vi "Create Enum Type Specialization.vi"(7 "error in":errorcluster, 9 "parameter name":string, 10 "enum reference in":refnum<vi>) -> (0 "error out":errorcluster, 2 "parameter type specialization output":T1, 3 "control reference out":refnum<vi>)   [LabVIEW 2020, in "Measurement Plugin Measurement Server.lvlib"]
uses:
  Measurement Plugin Measurement Server.lvlib
  TypeDefs/Parameter Type Specialization.ctl
  TypeDefs/Type Specialization.ctl
  TypeDefs/Type Specialization Key.ctl
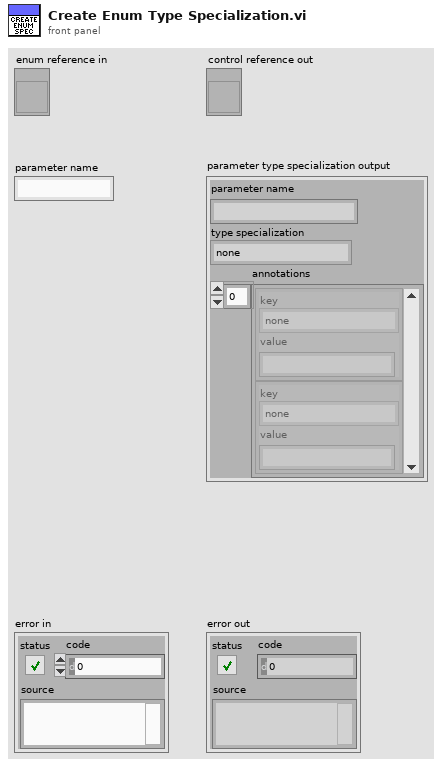
[diagram p1: front panel]
types:
  T1 = typedef "Measurement Plugin Measurement Server.lvlib/Parameter Type Specialization.ctl" = cluster{"parameter name":string, "type specialization":T2, "annotations":cluster{"key":T3, "value":string}[]}
  T2 = typedef "Measurement Plugin Measurement Server.lvlib/Type Specialization.ctl" = enum16{"none", "pin", "path", "enum", "ioresource"}
  T3 = typedef "Measurement Plugin Measurement Server.lvlib/Type Specialization Key.ctl" = enum16{"none", "pin.instrument_type", "enum.values", "ioresource.instrument_type"}
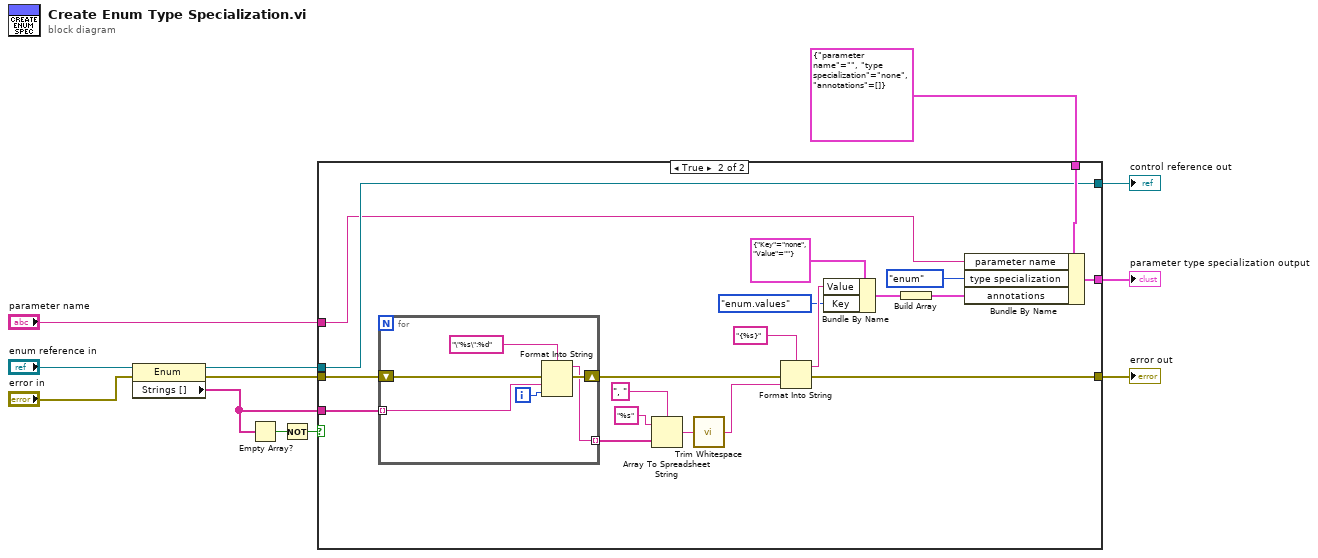
[diagram p0: block diagram]
diagram:
  n1 = property class="Enum"(reference="enum reference in", error in="error in") -> (reference out=w4:refnum<vi>, error out=w3:errorcluster, "Strings []"=w2:string[])
  n2 = Empty Array?(array=w2) -> (empty?=w8:bool)
  n3 = Not(x=w8) -> (.not. x?=w7:bool)
  n4 = case shown="True" w7 {
    tunnel: [w15 w34] -> w12
    tunnel: T1 {"parameter name"="", "type specialization"=enum."none", "annotations"=[]} ("Parameter Type Specialization Input") -> [w15 w32]
    tunnel: [w14 w27] -> w10
    tunnel: w2 -> [_ w19]
    tunnel: w4 -> [w13 w18]
    tunnel: [w13 w18] -> w9
    tunnel: w3 -> [w14 w17]
    tunnel: "parameter name" -> [_ w16]
    frame False {
    }
    frame True {
      n5 = for {
        tunnel: w19 -> [w40] mode=indexing
        shift-right: [w38] -> w28
        shift-left: w17 -> [w37]
        tunnel: [w36] -> w22 mode=indexing
        i -> [w39]
        n6 = Format Into String(format string="\"%s\":%d", error in=w37, w40, w39) -> (resulting string=w36:string, error out=w38:errorcluster)  [unwired: 1 in]
      }
      n7 = Array To Spreadsheet String(delimiter (Tab)=", ", array=w22, 3:"%s" ("format string")) -> (spreadsheet string=w21:string)
      n8 = call <vilib>:"Trim Whitespace.vi"("string"=w21) -> ("trimmed string"=w20:string)  [unwired: 1 in]
      n9 = Format Into String(format string="{%s}", error in=w28, w20) -> (resulting string=w30:string, error out=w27:errorcluster)  [unwired: 1 in]
      n10 = Bundle By Name(cluster=cluster{"Key":T3, "Value":string} {"Key"=enum."none", "Value"=""} ("input cluster"), "Value"=w30, "Key"=Type_Specialization_Key."enum.values") -> (w25:cluster{"Key":T3, "Value":string})
      n11 = Build Array(w25) -> (w26:cluster{"Key":T3, "Value":string}[])
      n12 = Bundle By Name(cluster=w32, "parameter name"=w16, "type specialization"=Type_Specialization."enum" ("Type Specialization"), "annotations"=w26) -> (w34:T1)
    }
  }
  "error out" <- w10
  "parameter type specialization output" <- w12
  "control reference out" <- w9
